vi "PID Control.vi"(1 "dt":dbl=0.001 format="%.3f", 2 "thetac":dbl[](array[numeric])=[-8.671875, -2.743055555555556, 0.22135416666666674], 3 "thetad":dbl[](array[numeric])=[2.0, 2.0, 2.0], 4 "PID gains":T1(array[cluster])=[{"proportional gain (Kc)"=1.0, "integral time (Ti, min)"=0.01, "derivative time (Td, min)"=0.0}] {"derivative time (Td, min)" format="%.3f"; "integral time (Ti, min)" format="%.3f"; "proportional gain (Kc)" format="%.3f"}) -> (0 "thetac'":dbl[](array[numeric])=[491.328125, 471.5625, 178.08593749999997])   [LabVIEW 2017]
uses:
  <vilib>/addons/control/pid/pid.llb/PID (DBL Array).vi
  <vilib>/addons/control/pid/NI_PID_pid.lvlib
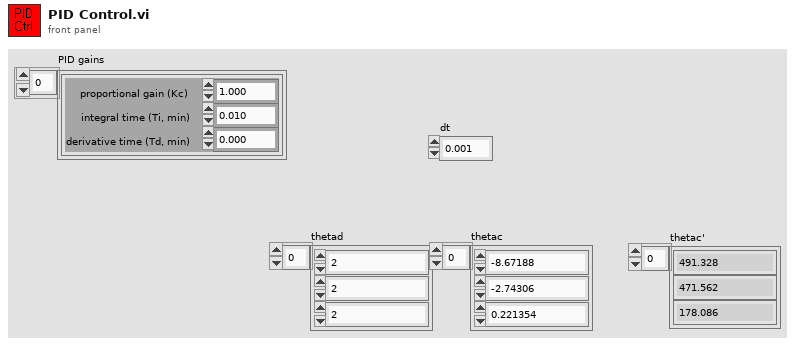
[diagram p1: front panel]
types:
  T1 = cluster{"proportional gain (Kc)":dbl, "integral time (Ti, min)":dbl, "derivative time (Td, min)":dbl}[]
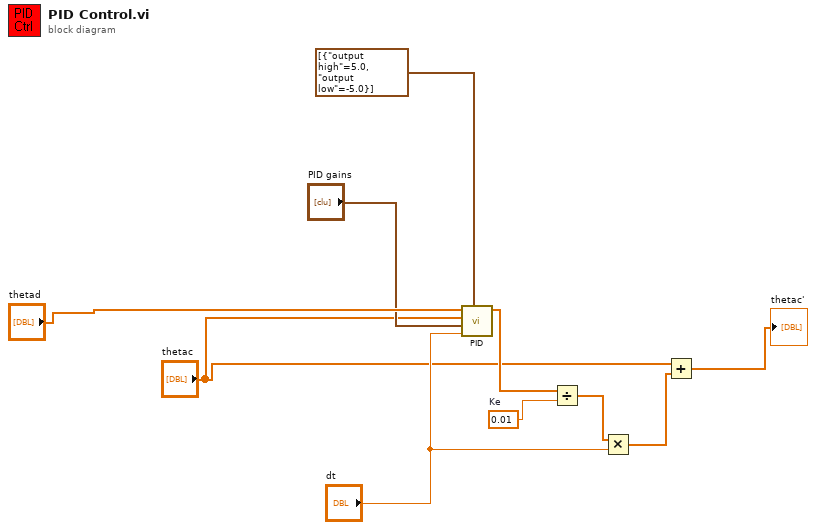
[diagram p0: block diagram]
diagram:
  w6 = 0.01  # Ke
  n1 = call-poly <vilib>:"PID.vi"("output range"=cluster{"output high":dbl, "output low":dbl}[] [{"output high"=5.0, "output low"=-5.0}], "dt (s)"="dt", "PID gains"="PID gains", "process variable"="thetac", "setpoint"="thetad") -> ("output"=w7:dbl[])  [unwired: 5 in, 1 out]
  n2 = Divide(x=w7, y=w6) -> (x/y=w5:dbl[])
  n3 = Multiply(x=w5, y="dt") -> (x*y=w3:dbl[])
  n4 = Add(x="thetac", y=w3) -> (x+y=→"thetac'":dbl[])
